vi "Get Image.vi"(8 "error in (no error)":errorcluster, 11 "Picam in":refnum<class "Picam.lvclass">) -> (0 "error out":errorcluster, 2 "Image":u16[][](array[numeric]), 3 "Picam out":refnum<class "Picam.lvclass">)   [LabVIEW 2019, in "Picam.lvclass"]
uses:
  Picam.lvclass
  Picam.lvclass/Picam.ctl
  picam32_LabView_SDK/PICam_lib/PICam.lvlib
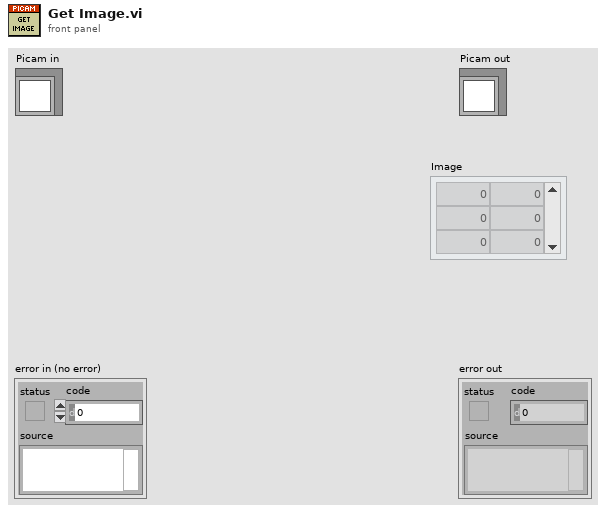
[diagram p1: front panel]
types:
  T1 = typedef "PICam.lvlib/DataAcquisitionResult.ctl" = cluster{"Bytes":u8[], "ReadoutCount":i64, "FramesPerReadout":i32, "Rois":T2[], "PixelBitDepth":i32, "TimeStampBitDepth":i32, "FrameTrackingBitDepth":i32, "GateTrackingBitDepth":i32, "ModulationTrackingBitDepth":i32}
  T2 = typedef "PicamRoi.ctl" = cluster{"x":i32, "width":i32, "x_binning":i32, "y":i32, "height":i32, "y_binning":i32}
  T3 = typedef "PICam.lvlib/PicamAcquisitionStatus.ctl" = cluster{"running":bool, "errors":T4, "readout_rate":dbl}
  T4 = typedef "PICam.lvlib/PicamAcquisitionErrorsMask.ctl" = enum8{"None", "DataLost", "ConnectionLost", "3", "DataNotArriving", "5", "6", "7", "ShutterOverheated", "9", "10", "11", "12", "13", "14", "15", "CameraFaulted"}
  T5 = typedef "PICam.lvlib/PicamAvailableData.ctl" = cluster{"initial_readout":u64, "readout_count":i64}
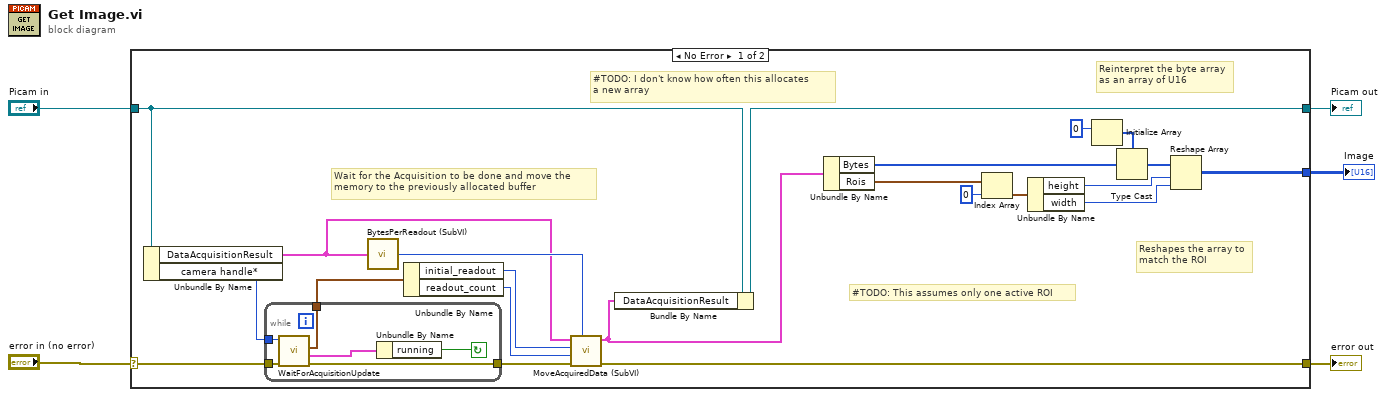
[diagram p0: block diagram]
diagram:
  n1 = case shown="No Error" "error in (no error)" {
    selector: "error in (no error)" -> [w27 w35]
    tunnel: [w22 w35] -> w4
    tunnel: [w17 w34] -> w2
    tunnel: "Picam in" -> [w25 w34]
    tunnel: [w8 _] -> w1
    frame No Error {
      # "Reshapes the array to\nmatch the ROI"
      # "Reinterpret the byte array\nas an array of U16"
      # "#TODO: This assumes only one active ROI"
      # "Wait for the Acquisition to be done and move the\nmemory to the previously allocated buffer"
      # "#TODO: I don't know how often this allocates\na new array"
      n2 = Unbundle By Name(w25) -> ("DataAcquisitionResult"=w20:T1, "camera handle*"=w24:u64)
      n3 = while {
        tunnel: w27 -> [w33]
        tunnel: [w32] -> w23
        tunnel: [w30] -> w26
        tunnel: w24 -> [w29]
        stop <- w31 continue-if-true
        n4 = call "WaitForAcquisitionUpdate.vi"("error in (no error)"=w33, "camera handle in"=w29) -> ("error out"=w32:errorcluster, "PicamAcquisitionStatus* status"=w28:T3, "PicamAvailableData* (available)"=w30:T5)  [unwired: 6 in, 1 out]
        n5 = Unbundle By Name(w28) -> ("running"=w31:bool)
      }
      n6 = call "BytesPerReadout (SubVI).vi"("DataAcquisitionBuffer in"=w20) -> ("Bytes/Readout >"=w21:i32)
      n7 = Unbundle By Name(w26) -> ("initial_readout"=w18:u64, "readout_count"=w19:i64)
      n8 = call "MoveAcquiredData (SubVI).vi"("Bytes/Readout >"=w21, "error in (no error)"=w23, "readout_count"=w19, "initial_readout*"=w18, "DataAcquisitionBuffer in"=w20) -> ("error out"=w22:errorcluster, "DataAcquisitionBuffer out"=w16:T1)  [unwired: 5 in]
      n9 = Bundle By Name(cluster=w25, "DataAcquisitionResult"=w16) -> (w17:refnum<class "Picam.lvclass">)
      n10 = Unbundle By Name(w16) -> ("Bytes"=w11:u8[], "Rois"=w15:T2[])
      n11 = Index Array(array=w15, index=0) -> (element=w13:T2)
      n12 = Unbundle By Name(w13) -> ("height"=w7:i32, "width"=w6:i32)
      n13 = Initialize Array(u16 0 ("element")) -> (w9:u16[])  [unwired: 1 in]
      n14 = Type Cast(type=w9, x=w11) -> (*(type *) &x=w12:u16[])
      n15 = Reshape Array(w12, w7, w6) -> (w8:u16[][])
    }
    frame Error {
    }
  }
  "error out" <- w4
  "Picam out" <- w2
  "Image" <- w1
